vi "Limit Testing for Unevenly Sampled Data.vi"() -> ()   [LabVIEW 2023]
doc: "Performs limit testing on unevenly sampled data. You might have unevenly sampled data in some applications, such as data sampled on a logarithmic scale.\n\nThis example uses the Limit Specification for Unevenly Sampled Data subVI. If you do not wire the dx and the x0 inputs, this VI accepts an array of X axis values at which your signal is sampled. It creates the limit at these X values. The example then uses the Limit Testing VI to compare the signal with the limits."
uses:
  <vilib>/measure/mamon.llb/Limit Testing Time.vi
  <vilib>/measure/NI_MAPro.lvlib
panel:
  out "test passed?":bool
  in  "Lower Limit":cluster{"X values":dbl[], "Y values":dbl[]}={"X values"=[6.0, 11.0, 16.0], "Y values"=[0.5, 0.4, 0.1]}
  in  "Upper Limit":cluster{"X values":dbl[], "Y values":dbl[]}={"X values"=[6.0, 11.0, 16.0], "Y values"=[1.0, 0.8, 0.5]}
  out "Limit Test":T1(graph)
  in  "X Values for Signal":dbl[](array[numeric])=[4.5, 6.0, 6.7, 9.0, 11.0, 13.0]
  in  "Y values for Signal":dbl[](array[numeric])=[0.9, 0.85, 0.6, 0.8, 0.5, 0.5]
  # "Overview: This example shows how to run a limit test on unevenly sampled data.\nRequirements: LabVIEW Full Development System\nInstructions: \n1. Run the VI.  \n2. Change the Y values for Signal to contain values above the Upper Limit or below the Lower Limit and run the VI again. The limit test should fail."
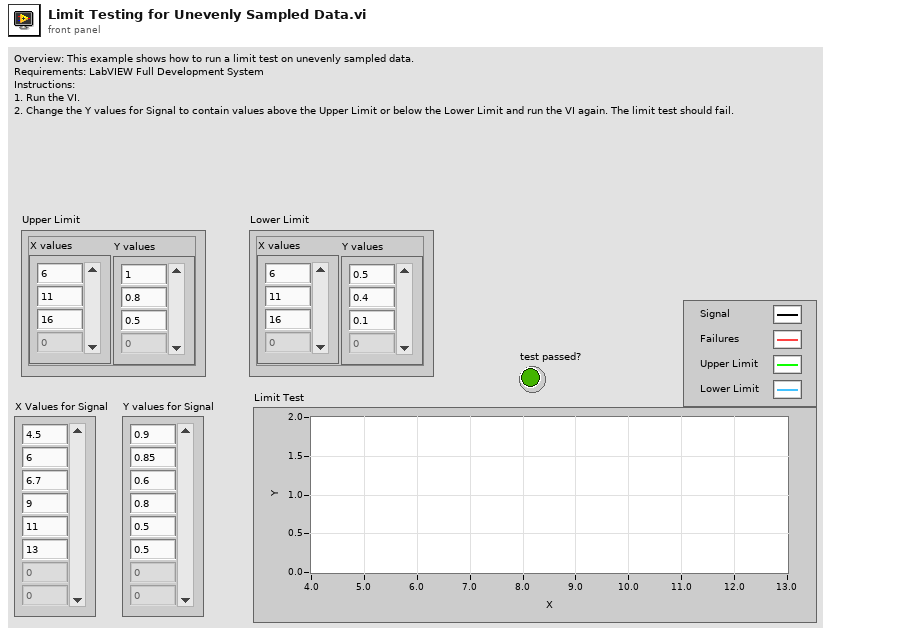
[diagram p1: front panel]
types:
  T1 = cluster{"X Values for Signal":dbl[], "Y":dbl[]}[]
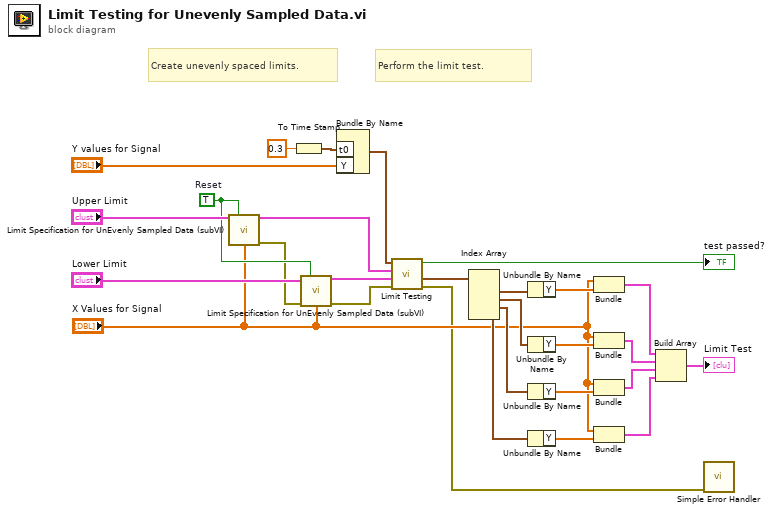
[diagram p0: block diagram]
diagram:
  w5 = TRUE  # Reset
  # "Perform the limit test."
  # "Create unevenly spaced limits."
  n1 = call "Limit Specification for UnEvenly Sampled Data (subVI).vi"("Specification Cluster"="Upper Limit", "reset"=w5, "X Values for Signal"="X Values for Signal") -> ("Limit"=w11:cluster{"x0":dbl, "dx":dbl, "Y":dbl[]}, "error out"=w2:errorcluster)  [unwired: 11 in]
  n2 = To Time Stamp(1:0.3) -> (0:w9:timestamp)
  n3 = call "Limit Specification for UnEvenly Sampled Data (subVI).vi"("Specification Cluster"="Lower Limit", "reset"=w5, "error in (no error)"=w2, "X Values for Signal"="X Values for Signal") -> ("Limit"=w10:cluster{"x0":dbl, "dx":dbl, "Y":dbl[]}, "error out"=w1:errorcluster)  [unwired: 10 in]
  n4 = Bundle By Name("t0"=w9, "Y"="Y values for Signal") -> (w23:waveform(dbl))  [unwired: 1 in]
  n5 = call-poly <vilib>:"Limit Testing.vi"("error in (no error)"=w1, "lower limit"=w10, "upper limit"=w11, "signal in"=w23) -> ("error out"=w3:errorcluster, "output values"=w22:waveform(dbl)[], "test passed?"=→"test passed?":bool)  [unwired: 2 in, 3 out]
  n6 = Index Array(array=w22) -> (element #1=w21:waveform(dbl), element #2=w8:waveform(dbl), element #3=w7:waveform(dbl), element #4=w6:waveform(dbl))  [unwired: 4 in]
  n7 = Unbundle By Name(w21) -> ("Y"=w20:dbl[])
  n8 = Unbundle By Name(w8) -> ("Y"=w19:dbl[])
  n9 = Unbundle By Name(w7) -> ("Y"=w18:dbl[])
  n10 = Unbundle By Name(w6) -> ("Y"=w17:dbl[])
  n11 = Bundle("X Values for Signal"="X Values for Signal", "Y"=w20) -> (w26:cluster{"X Values for Signal":dbl[], "Y":dbl[]})  [unwired: 1 in]
  n12 = Bundle("X Values for Signal"="X Values for Signal", "Y"=w19) -> (w25:cluster{"X Values for Signal":dbl[], "Y":dbl[]})  [unwired: 1 in]
  n13 = Bundle("X Values for Signal"="X Values for Signal", "Y"=w18) -> (w24:cluster{"X Values for Signal":dbl[], "Y":dbl[]})  [unwired: 1 in]
  n14 = Bundle("X Values for Signal"="X Values for Signal", "Y"=w17) -> (w15:cluster{"X Values for Signal":dbl[], "Y":dbl[]})  [unwired: 1 in]
  n15 = Build Array(w26, w25, w24, w15) -> (→"Limit Test":T1)
  n16 = call <vilib>:"Simple Error Handler.vi"("error in (no error)"=w3) -> ()  [unwired: 4 in, 5 out]
